vi "Time stamp to SQL string.vi"(2 "SQL formatting?":bool, 3 "time stamp":timestamp) -> (0 "SQL format date-time string":string, 1 "Seconds Since 1904":i64)   [LabVIEW 2010, in "SQL project lib.lvlib"]
uses:
  SQL project lib.lvlib
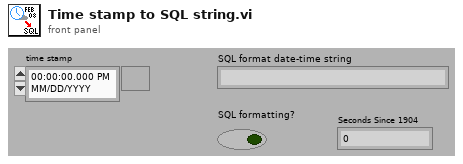
[diagram p1: front panel]
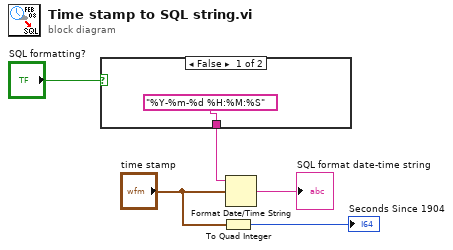
[diagram p0: block diagram]
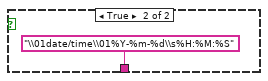
[diagram p2: hidden frame]
diagram:
  n1 = case shown="False" "SQL formatting?" {
    tunnel: ["%Y-%m-%d %H:%M:%S" ("time format string (%c)") "\\01date/time\\01%Y-%m-%d\\s%H:%M:%S" ("time format string (%c)")] -> w5
    frame False {
    }
    frame True {
    }
  }
  n2 = To Quad Integer(1:"time stamp") -> (0:→"Seconds Since 1904":i64)
  n3 = Format Date/Time String(time format string (%c)=w5, seconds (now)="time stamp") -> (date/time string=→"SQL format date-time string":string)  [unwired: 1 out]
